vi "Format FTT String.vi"(0 "Num in":dbl, 1 "Use Rate?":bool) -> (5 "Num out":string)   [LabVIEW 2014]
panel:
  out "error out":errorcluster
  in  "error in":errorcluster
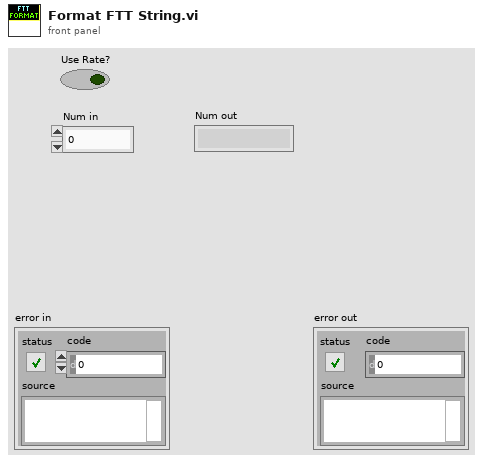
[diagram p1: front panel]
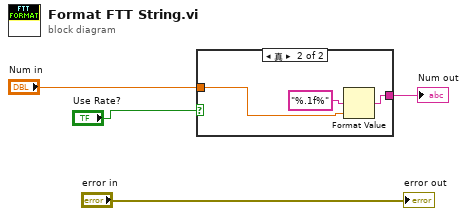
[diagram p0: block diagram]
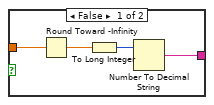
[diagram p2: hidden frame]
diagram:
  n1 = case shown="真" "Use Rate?" {
    tunnel: "Num in" -> [w7 w9]
    tunnel: [w5 w10] -> w2
    frame False {
      n2 = Round Toward -Infinity(1:w7) -> (0:w8:dbl)
      n3 = To Long Integer(number=w8) -> (32bit integer=w6:i32)
      n4 = Number To Decimal String(number=w6) -> (decimal integer string=w5:string)  [unwired: 1 in]
    }
    frame True {
      n5 = Format Value(format string="%.1f%", value (0)=w9) -> (output string=w10:string)  [unwired: 1 in]
    }
  }
  "Num out" <- w2
  "error out" <- "error in"
